vi "Get Array of Elements.vi"(8 "error in (no error)":errorcluster, 10 "Tag Name":string, 11 "Refnum in":refnum<k20>) -> (0 "error out":errorcluster, 2 "Array Of Elements":refnum<k20>[](array[refnum]), 3 "Refnum out":refnum<k20>)   [LabVIEW 2020]
uses:
  <resource>/objmgr/DOMUserDefRef.rc
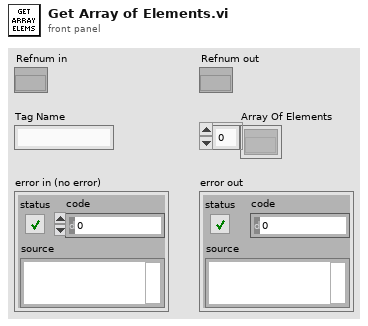
[diagram p1: front panel]
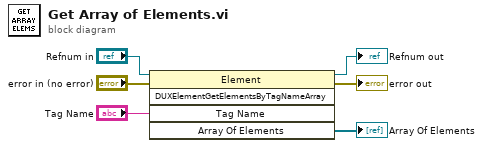
[diagram p0: block diagram]
diagram:
  n1 = invoke class="Element" method="DUXElementGetElementsByTagNameArray"(reference="Refnum in", error in="error in (no error)", "Tag Name"="Tag Name") -> (reference out=→"Refnum out":refnum<k20>, error out=→"error out":errorcluster, "Array Of Elements"=→"Array Of Elements":refnum<k20>[])  [unwired: 2 in, 2 out]
